vi "sql-delete_vcmd.vi"(0 "input-IP":string="dg-sql-01.luxshare.com.cn", 1 "input-user":string="htpsuser\n", 2 "input-psw":string="htps'songyy", 3 "input-db":string="HTPSDB", 4 "操作模式":T1(ring)=enum."删除数据", 5 "列名":string[](array[string]), 6 "表名":string="vcmd", 7 "数据类型":string[](array[combo]), 9 "主键":string, 11 "限定条件":string="where CmdType='LR Q to S 4X'") -> (12 "错误类型":string, 15 "status":bool)   [LabVIEW 2011]
panel:
  out "字符串":string
  out "错误输出 1":errorcluster
  out "code":i32
  out "错误输出":errorcluster
  in  "ADODB._Recordset":refnum<k7>
  in  "ADODB._Connection":refnum<k7>
  # "输       入"
  # "输       出"
  # "基本信息\n（）"
  # "创建表、添加表列、删除表列时需要填写\n\n创建的表的列名称、添加的列的名称、删除的列的名称\n\n后面的数据类型，为创建表、添加列时才需要指定的，定义列的数据类型"
  # "状态灯，False表示操作失败，True表示操作成功"
  # "错误类型"
  # "改变操作时需要修改的信息"
  # "操作模式：创建表\n                  删除表\n                  添加表列\n                  删除表列"
  # "表名"
  # "主键，只有在创建表的时候才需要填写，指定创建表列中的一列为主键"
  # "创建表、添加表列、删除表列时需要选择\n\n创建的表所包含的列数、添加的列数、删除的列数"
  # "删除用户时需要填写，利用条件查找需要删除的用户行"
  # "error:\n-2147217843 登陆失败： 。\n-2147467259 要访问的数据库不存在\n-2146825267 没有数据    。\n-2146824584 对象关闭时，不允许操作\n-2147217865 表名不存在 。\n-2147467259 服务器连接失败 。"
  # "error:\n-2147217900 所创建的表已经存在\n-2147217900 该列不存在"
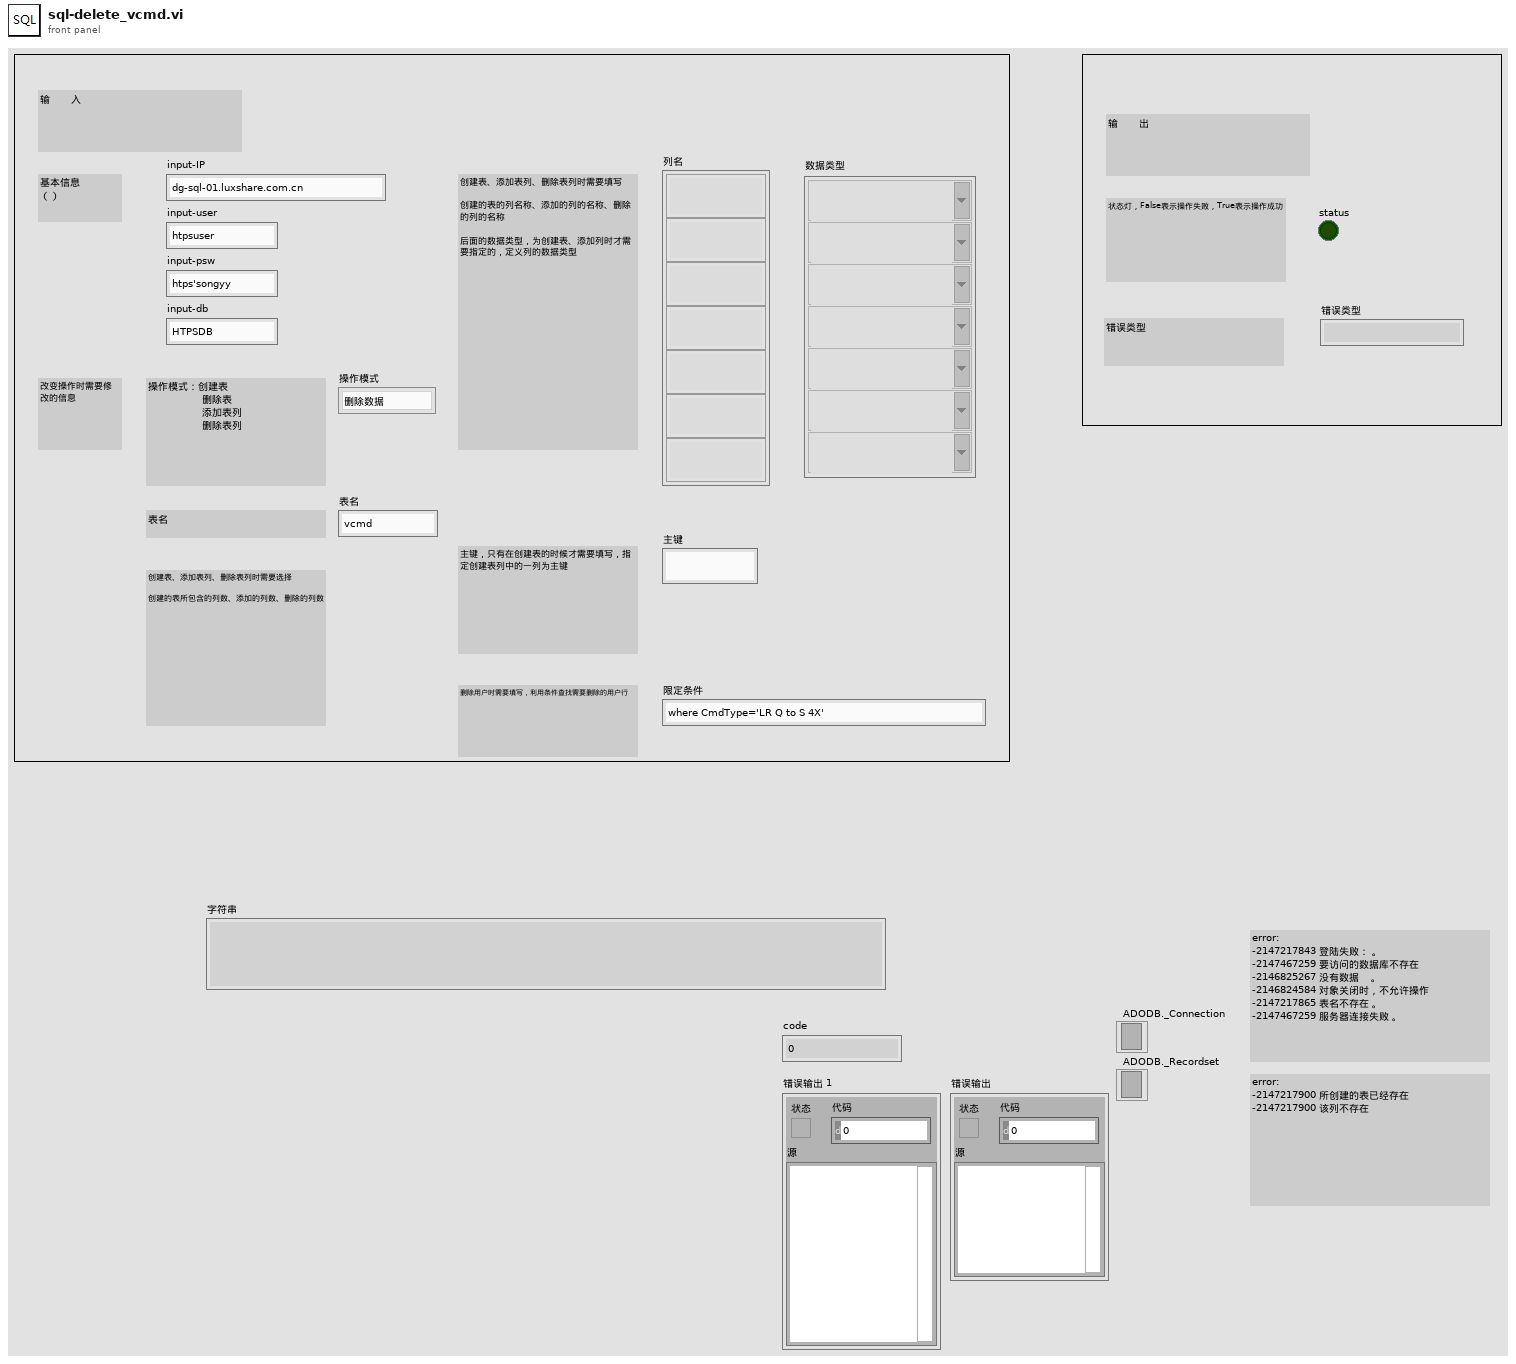
[diagram p1: front panel]
types:
  T1 = enum16{"", "创建表", "删除表", "添加表列", "删除表列", "添加数据", "删除数据"}
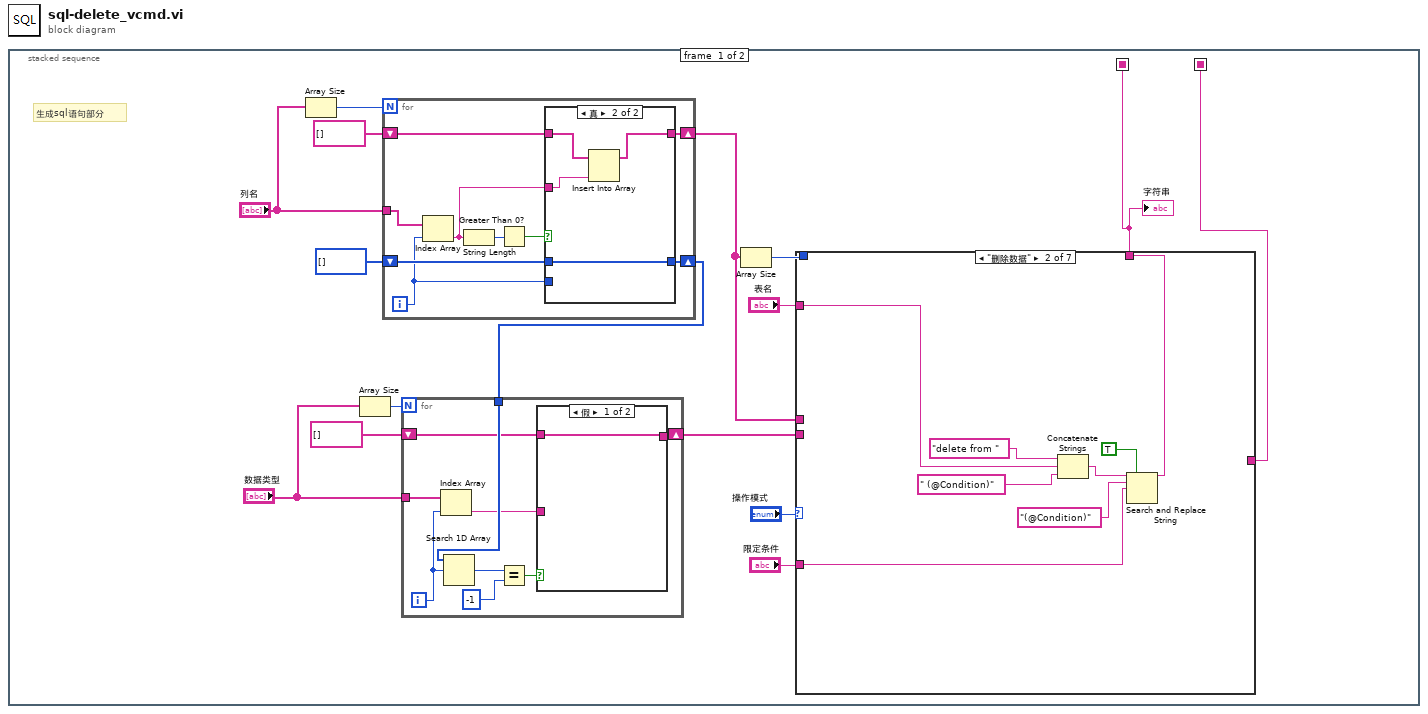
[diagram p0: block diagram]
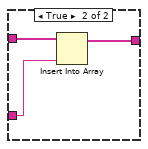
[diagram p2: hidden frame]
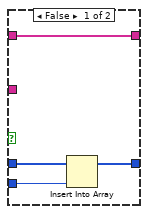
[diagram p3: hidden frame]
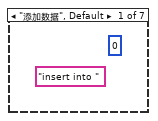
[diagram p4: hidden frame]
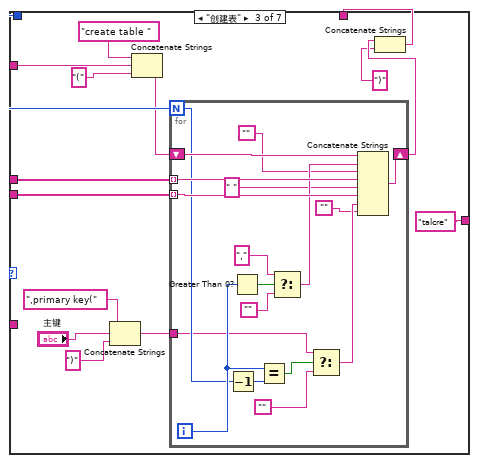
[diagram p5: hidden frame]
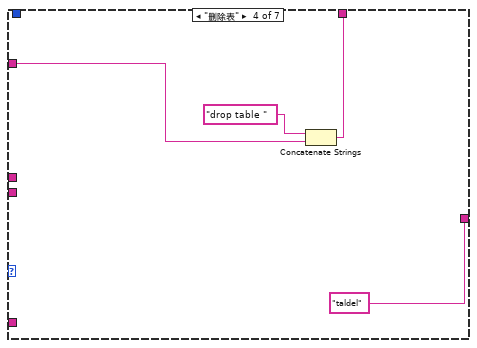
[diagram p6: hidden frame]
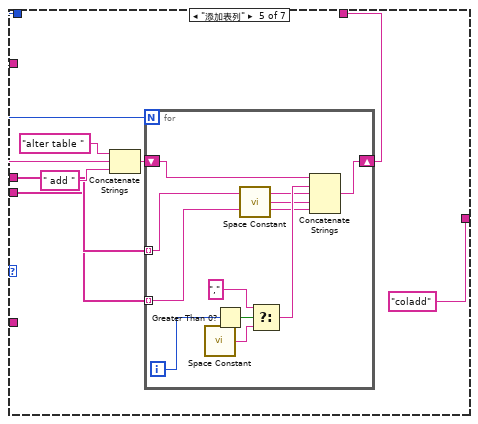
[diagram p7: hidden frame]
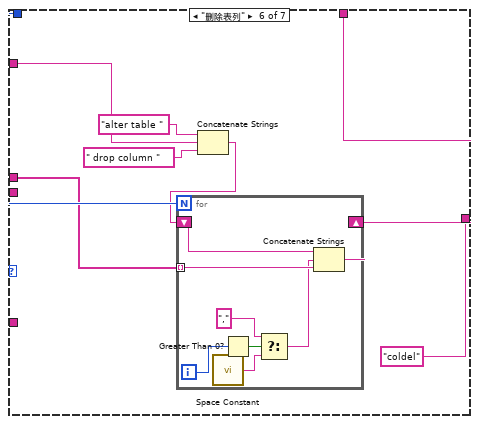
[diagram p8: hidden frame]
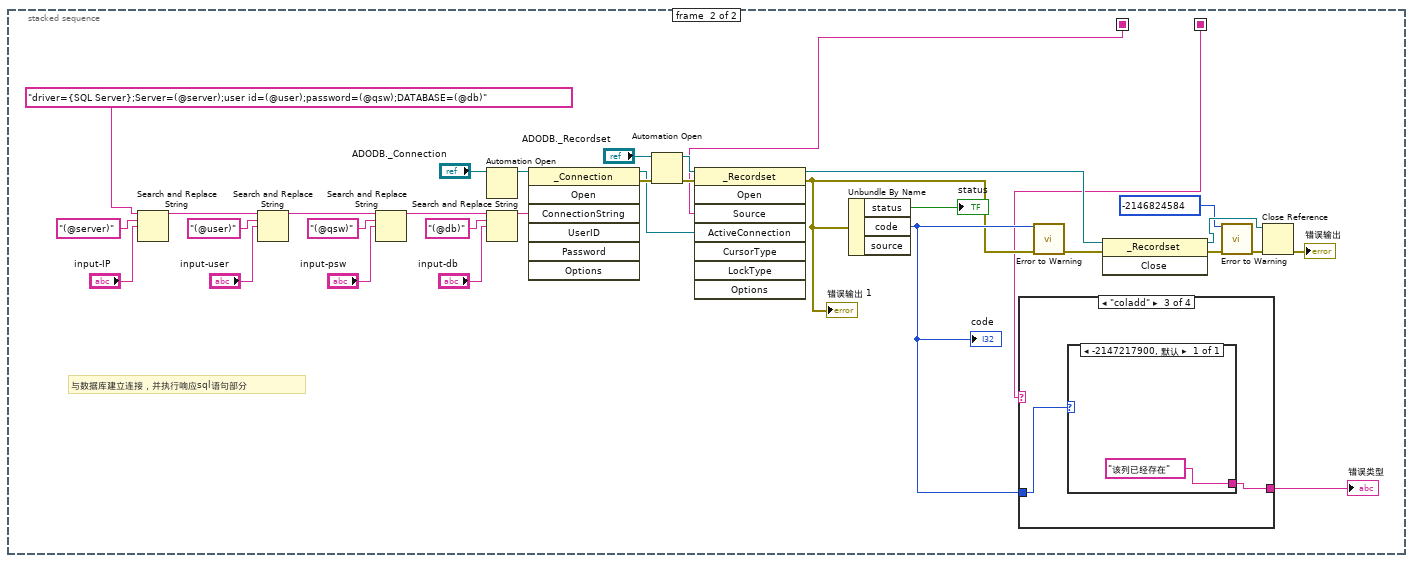
[diagram p10: hidden frame]
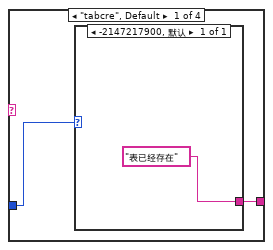
[diagram p11: hidden frame]
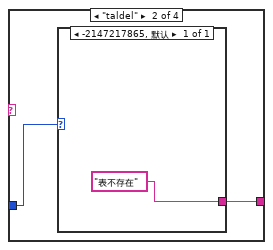
[diagram p12: hidden frame]
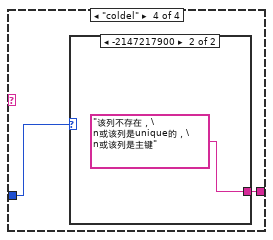
[diagram p13: hidden frame]
diagram:
  n1 = stacked-sequence {
    seq-local: [w1 _] -> [_ w129]
    seq-local: [w2 _] -> [_ w128]
    frame #0 {
      # "生成sql语句部分"
      n2 = Array Size(array="列名") -> (size(s)=w14:i32)
      n3 = Array Size(array="数据类型") -> (size(s)=w11:i32)
      n4 = for {
        N: w14 -> [_]
        tunnel: "列名" -> [w38]
        shift-right: [w33] -> w5
        shift-left: string[] [] -> [w34]
        shift-right: [w30] -> w9
        shift-left: i32[] [] -> [w32]
        i -> [w31]
        n5 = Index Array(array=w38, index=w31) -> (element=w35:string)
        n6 = String Length(string=w35) -> (length=w37:i32)
        n7 = Greater Than 0?(x=w37) -> (x > 0?=w36:bool)
        n8 = case shown="真" w36 {
          tunnel: w35 -> [_ w44]
          tunnel: w34 -> [w42 w46]
          tunnel: [w42 w45] -> w33
          tunnel: w32 -> [w41 w43]
          tunnel: w31 -> [w40 _]
          tunnel: [w39 w43] -> w30
          frame False {
            n9 = Insert Into Array(array=w41, new element=w40) -> (w39:i32[])  [unwired: 1 in]
          }
          frame True {
            n10 = Insert Into Array(array=w46, new element=w44) -> (w45:string[])  [unwired: 1 in]
          }
        }
      }
      n11 = for {
        N: w11 -> [_]
        shift-right: [w17] -> w3
        shift-left: string[] [] -> [w18]
        tunnel: "数据类型" -> [w22]
        tunnel: w9 -> [w25]
        i -> [w21]
        n12 = Index Array(array=w22, index=w21) -> (element=w19:string)
        n13 = Search 1D Array(1D array=w25, element=w21) -> (index of element=w24:i32)  [unwired: 1 in]
        n14 = Equal?(x=w24, y=-1) -> (x = y?=w20:bool)
        n15 = case shown="假" w20 {
          tunnel: w19 -> [_ w27]
          tunnel: w18 -> [w26 w29]
          tunnel: [w26 w28] -> w17
          frame False {
          }
          frame True {
            n16 = Insert Into Array(array=w29, new element=w27) -> (w28:string[])  [unwired: 1 in]
          }
        }
      }
      n17 = Array Size(array=w5) -> (size(s)=w6:i32)
      n18 = case shown="\"删除数据\"" "操作模式" {
        tunnel: "表名" -> [_ w53 w67 w90 w98 w117 _]
        tunnel: [_ w50 w55 w89 w93 w112 _] -> w1
        tunnel: w6 -> [_ _ w69 _ w99 w115 _]
        tunnel: w5 -> [_ _ w56 _ w96 w113 _]
        tunnel: w3 -> [_ _ w65 _ w92 _ _]
        tunnel: [_ _ "talcre" "taldel" "coladd" "coldel" _] -> w2
        tunnel: "限定条件" -> [_ w47 _ _ _ _ _]
        frame "添加数据", Default {
          (unwired) "insert into "
          (unwired) 0
        }
        frame "删除数据" {
          n19 = Concatenate Strings("delete from ", w53, " (@Condition)") -> (w51:string)
          n20 = Search and Replace String(replace all?=TRUE ("替换全部？(F)"), input string=w51, search string="(@Condition)" ("搜索字符串"), replace string=w47) -> (result string=w50:string)  [unwired: 4 in, 3 out]
        }
        frame "创建表" {
          n21 = Concatenate Strings(",primary key(", "主键", ")") -> (w60:string)
          n22 = Concatenate Strings("create table ", w67, "(" ("字符串")) -> (w64:string)
          n23 = for {
            N: w69 -> [w78]
            tunnel: w56 -> [w87] mode=indexing
            tunnel: w65 -> [w86] mode=indexing
            shift-right: [w73] -> w59
            shift-left: w64 -> [w82]
            tunnel: w60 -> [w76]
            i -> [w80]
            n24 = Decrement(x=w78) -> (x-1=w79:i32)
            n25 = Greater Than 0?(x=w80) -> (x > 0?=w85:bool)
            n26 = Equal?(x=w80, y=w79) -> (x = y?=w77:bool)
            n27 = Select(t=",", s=w85, f="") -> (s? t:f=w81:string)
            n28 = Select(t=w76, s=w77, f="") -> (s? t:f=w74:string)
            n29 = Concatenate Strings(w82, w81, "", w87, " ", w86, w74, "") -> (w73:string)
          }
          n30 = Concatenate Strings(w59, ")") -> (w55:string)
        }
        frame "删除表" {
          n31 = Concatenate Strings("drop table ", w90) -> (w89:string)
        }
        frame "添加表列" {
          n32 = Concatenate Strings("alter table ", w98, " add ") -> (w95:string)
          n33 = for {
            N: w99 -> [_]
            tunnel: w96 -> [w104] mode=indexing
            shift-right: [w103] -> w93
            shift-left: w95 -> [w110]
            tunnel: w92 -> [w102] mode=indexing
            i -> [w106]
            n34 = call <vilib>:"Space Constant.vi"() -> ("String"=w107:string)
            n35 = Greater Than 0?(x=w106) -> (x > 0?=w109:bool)
            n36 = call <vilib>:"Space Constant.vi"() -> ("String"=w101:string)
            n37 = Select(t=",", s=w109, f=w107) -> (s? t:f=w105:string)
            n38 = Concatenate Strings(w110, w105, w104, w101, w102) -> (w103:string)
          }
        }
        frame "删除表列" {
          n39 = Concatenate Strings("alter table ", w117, " drop column ") -> (w114:string)
          n40 = for {
            N: w115 -> [_]
            tunnel: w113 -> [w125] mode=indexing
            shift-right: [w119] -> w112
            shift-left: w114 -> [w126]
            i -> [w120]
            n41 = call <vilib>:"Space Constant.vi"() -> ("String"=w124:string)
            n42 = Greater Than 0?(x=w120) -> (x > 0?=w122:bool)
            n43 = Select(t=",", s=w122, f=w124) -> (s? t:f=w121:string)
            n44 = Concatenate Strings(w126, w121, w125) -> (w119:string)
          }
        }
        frame "" {
        }
      }
      "字符串" <- w1
    }
    frame #1 {
      # "与数据库建立连接，并执行响应sql语句部分"
      n45 = Search and Replace String(input string="driver={SQL Server};Server=(@server);user id=(@user);password=(@qsw);DATABASE=(@db)" ("ConnectionString"), search string="(@server)" ("搜索字符串"), replace string="input-IP") -> (result string=w134:string)  [unwired: 5 in, 3 out]
      n46 = Search and Replace String(input string=w134, search string="(@user)" ("搜索字符串"), replace string="input-user") -> (result string=w137:string)  [unwired: 5 in, 3 out]
      n47 = Search and Replace String(input string=w137, search string="(@qsw)" ("搜索字符串"), replace string="input-psw") -> (result string=w140:string)  [unwired: 5 in, 3 out]
      n48 = Automation Open(Automation Refnum="ADODB._Connection") -> (Automation Refnum=w130:refnum<k7>)  [unwired: 3 in, 1 out]
      n49 = Search and Replace String(input string=w140, search string="(@db)" ("搜索字符串"), replace string="input-db") -> (result string=w144:string)  [unwired: 5 in, 3 out]
      n50 = invoke class="_Connection" method="Open"(reference=w130, "ConnectionString"=w144) -> (reference out=w146:refnum<k7>, error out=w148:errorcluster)  [unwired: 5 in, 5 out]
      n51 = Automation Open(error in (no error)=w148, Automation Refnum="ADODB._Recordset") -> (Automation Refnum=w147:refnum<k7>, error out=w149:errorcluster)  [unwired: 2 in]
      n52 = invoke class="_Recordset" method="Open"(reference=w147, error in=w149, "Source"=w129, "ActiveConnection"=w146) -> (reference out=w156:refnum<k7>, error out=w157:errorcluster)  [unwired: 4 in, 6 out]
      "错误输出 1" <- w157
      n53 = Unbundle By Name(w157) -> ("status"=→"status":bool, "code"=w159:i32)  [unwired: 1 out]
      "code" <- w159
      n54 = case shown="\"coladd\"" w128 {
        tunnel: w159 -> [w161 w164 w167 w170]
        tunnel: [w160 w163 w166 w169] -> w158
        frame "tabcre", Default {
          n55 = case shown="-2147217900, 默认" w161 {
            tunnel: ["表已经存在"] -> w160
            frame -2147217900, Default {
            }
          }
        }
        frame "taldel" {
          n56 = case shown="-2147217865, 默认" w164 {
            tunnel: ["表不存在"] -> w163
            frame -2147217865, Default {
            }
          }
        }
        frame "coladd" {
          n57 = case shown="-2147217900, 默认" w167 {
            tunnel: ["该列已经存在"] -> w166
            frame -2147217900, Default {
            }
          }
        }
        frame "coldel" {
          n58 = case shown="-2147217900" w170 {
            tunnel: [_ "该列不存在，\n或该列是unique的，\n或该列是主键"] -> w169
            frame 0, Default {
            }
            frame -2147217900 {
            }
          }
        }
      }
      "错误类型" <- w158
      n59 = call <vilib>:"Error to Warning.vi"("1st Error to Convert"=w159, "error in"=w157) -> ("warning out"=w150:errorcluster)  [unwired: 13 in]
      n60 = invoke class="_Recordset" method="Close"(reference=w156, error in=w150) -> (reference out=w154:refnum<k7>, error out=w151:errorcluster)  [unwired: 1 in, 1 out]
      n61 = call <vilib>:"Error to Warning.vi"("1st Error to Convert"=-2146824584, "error in"=w151) -> ("warning out"=w155:errorcluster)  [unwired: 13 in]
      n62 = Close Reference(reference=w154, error in (no error)=w155) -> (error out=→"错误输出":errorcluster)
    }
  }
